vi "Import Pitch Calibration Data [Open Loop].vi"(8 "Error In":errorcluster, 11 "Pitch Data Ref":refnum<vi>) -> (0 "Error Out":errorcluster)   [LabVIEW 2017]
uses:
  Pitch Array 1.ctl
  <vilib>/Utility/file.llb/Read Delimited Spreadsheet (DBL).vi
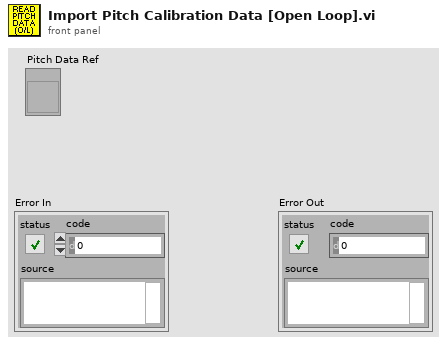
[diagram p1: front panel]
types:
  T1 = typedef "Pitch Array 1.ctl" = cluster{"Array":dbl[][], "Operation":bool}
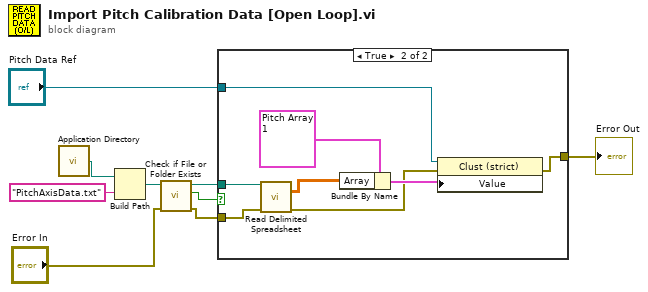
[diagram p0: block diagram]
diagram:
  n1 = call <vilib>:"Application Directory.vi"() -> ("Application Directory"=w7:path)
  n2 = Build Path(base path=w7, name or relative path="PitchAxisData.txt") -> (appended path=w5:path)
  n3 = call <vilib>:"Check if File or Folder Exists.vi"("error in (no error)"="Error In", "path"=w5) -> ("error out"=w1:errorcluster, "file or folder exists?"=w3:bool, "dup path"=w4:path)  [unwired: 7 in]
  n4 = case shown="True" w3 {
    tunnel: [w10 w18] -> w9
    tunnel: "Pitch Data Ref" -> [_ w17]
    tunnel: w4 -> [_ w13]
    tunnel: w1 -> [w10 w12]
    frame False {
    }
    frame True {
      n5 = call-poly <vilib>:"Read Delimited Spreadsheet.vi"("file path (dialog if empty)"=w13, "error in (no error)"=w12) -> ("all rows"=w16:dbl[][], "error out"=w11:errorcluster)  [unwired: 8 in, 4 out]
      n6 = Bundle By Name(cluster=T1 {"Array"=[[80.0, 0.9, 1.0, 1.0, 1.0, 1.0, 1.0, 1.0, 1.0], [70.0, 0.96, 0.0, 0.0, 0.0, 0.0, 0.0, 0.0, 0.0], [60.0, 1.08, 0.0, 0.0, 0.0, 0.0, 0.0, 0.0, 0.0], [50.0, 1.25, 0.0, 0.0, 0.0, 0.0, 0.0, 0.0, 0.0], [40.0, 1.44, 0.0, 0.0, 0.0, 0.0, 0.0, 0.0, 0.0], [30.0, 1.68, 0.0, 0.0, 0.0, 0.0, 0.0, 0.0, 0.0], [20.0, 1.91, 0.0, 0.0, 0.0, 0.0, 0.0, 0.0, 0.0], [10.0, 2.19, 0.0, 0.0, 0.0, 0.0, 0.0, 0.0, 0.0], [0.0, 2.47, 0.0, 0.0, 0.0, 0.0, 0.0, 0.0, 0.0], [-10.0, 2.73, 0.0, 0.0, 0.0, 0.0, 0.0, 0.0, 0.0], [-20.0, 3.01, 0.0, 0.0, 0.0, 0.0, 0.0, 0.0, 0.0], [-30.0, 3.3, 0.0, 0.0, 0.0, 0.0, 0.0, 0.0, 0.0], [-40.0, 3.5, 0.0, 0.0, 0.0, 0.0, 0.0, 0.0, 0.0], [-50.0, 3.72, 0.0, 0.0, 0.0, 0.0, 0.0, 0.0, 0.0], [-60.0, 3.92, 0.0, 0.0, 0.0, 0.0, 0.0, 0.0, 0.0], [-70.0, 4.05, 0.0, 0.0, 0.0, 0.0, 0.0, 0.0, 0.0], [-80.0, 4.11, 0.0, 0.0, 0.0, 0.0, 0.0, 0.0, 0.0]], "Operation"=FALSE} ("Pitch Calib"), "Array"=w16) -> (w15:T1)
      n7 = property class="Clust (strict)"(reference=w17, error in=w11, "Value"=w15) -> (error out=w18:errorcluster)  [unwired: 1 out]
    }
  }
  "Error Out" <- w9
